vi "Get List Image With Parameters.vi"(0 "Template in":refnum<class "MetaDataObj.lvclass">, 1 "Img Width":u32=230, 3 "DNL_Point":T1={"Horizontal"=-1, "Vertical"=-1}, 5 "Background Color":u32(colorbox)=16777215, 9 "Text Color":u32(colorbox), 11 "error in (no error)":errorcluster, 12 "Highlight?":bool, 13 "Underline Link?":bool) -> (4 "Template out":refnum<class "MetaDataObj.lvclass">, 6 "Image":picture, 10 "End of Desc Character":i32, 14 "Hovering Over Link?":bool, 15 "error out":errorcluster)   [LabVIEW 2016, in "MetaDataObj.lvclass"]
uses:
  <resource>/dialog/NewProjectWizard/MetaDataObj/MetaDataObj.lvclass
  <vilib>/Utility/miscctls.llb/LVPoint32TypeDef.ctl
  <resource>/dialog/NewProjectWizard/MetaDataObj/Accessors/Read Description.vi
  <resource>/dialog/NewProjectWizard/MetaDataObj/Accessors/Read Title.vi
  <resource>/dialog/NewProjectWizard/MetaDataObj/Accessors/Read Icon.vi
  <resource>/dialog/NewProjectWizard/MetaDataObj/Accessors/Read Documentation Path.vi
  <resource>/dialog/NewProjectWizard/MetaDataObj/Accessors/Read Filters.vi
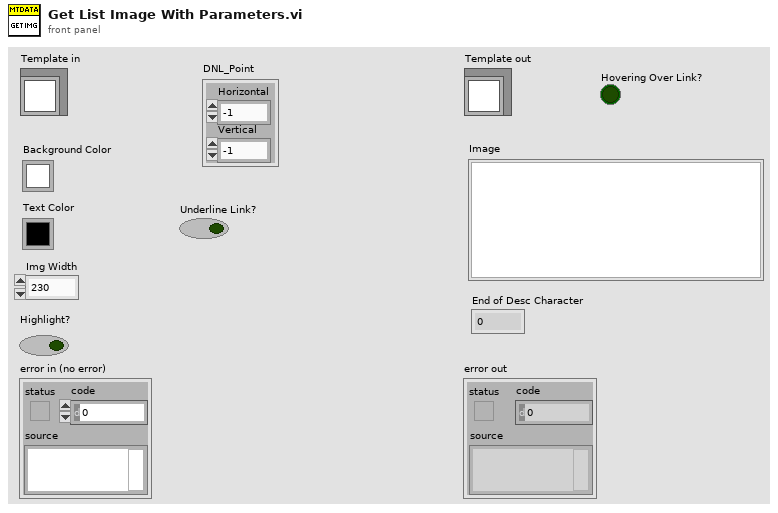
[diagram p1: front panel]
types:
  T1 = typedef "LVPoint32TypeDef.ctl" = cluster{"Horizontal":i32, "Vertical":i32}
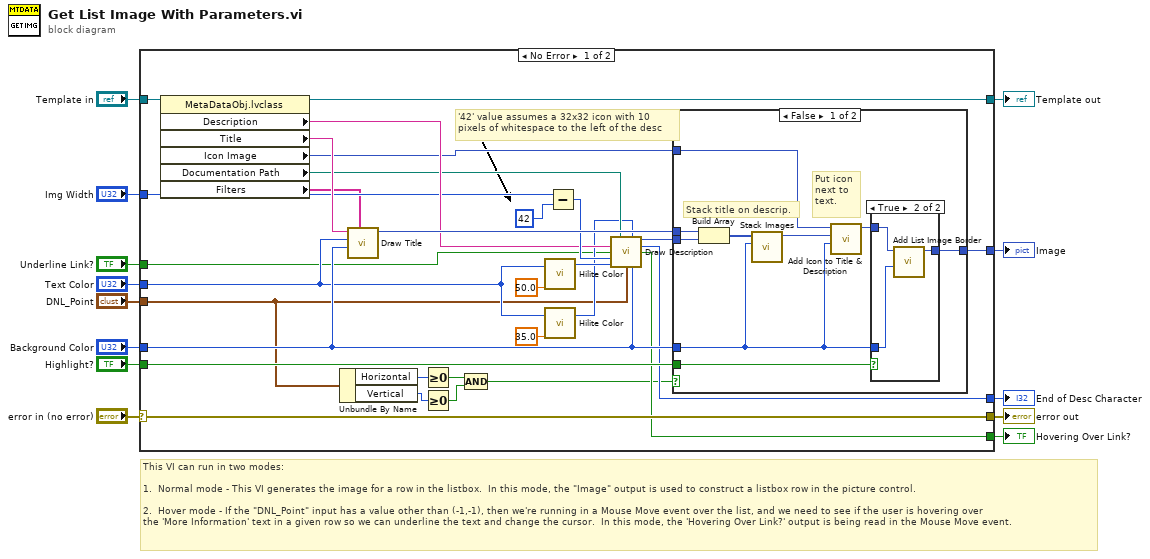
[diagram p0: block diagram]
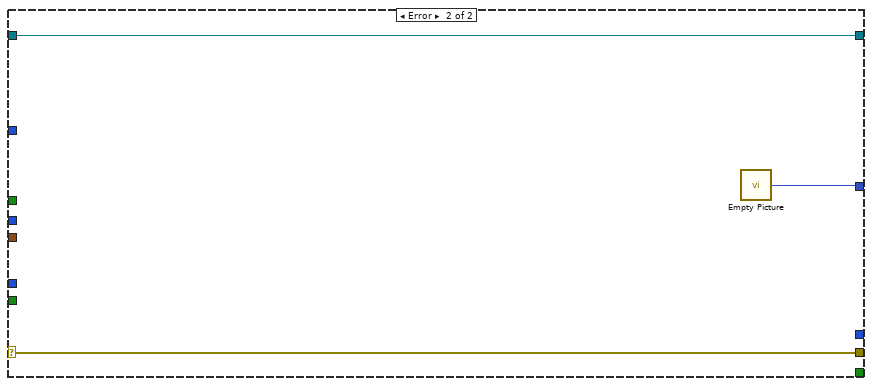
[diagram p4: hidden frame]
diagram:
  # "This VI can run in two modes:\n\n1.  Normal mode - This VI generates the image for a row in the listbox.  In this mode, the \"Image\" output is used to construct a listbox row in the picture control.\n\n2.  Hover mode - If the \"DNL_Point\" input has a value other than (-1,-1), then we're running in a Mouse Move event over the list, and we need to see if the user is hovering over\nthe 'More Information' text in a given row so we can underline the text and change the cursor.  In this mode, the 'Hovering Over Link?' output is being read in the Mouse Move event."
  n1 = case shown="No Error" "error in (no error)" {
    selector: "error in (no error)" -> [w43 w59]
    tunnel: [w43 w59] -> w12
    tunnel: [w33 w58] -> w10
    tunnel: "Template in" -> [w40 w58]
    tunnel: [w36 w57] -> w9
    tunnel: "Img Width" -> [w32 _]
    tunnel: "Text Color" -> [w27 _]
    tunnel: "Background Color" -> [w31 _]
    tunnel: "Highlight?" -> [w30 _]
    tunnel: [w25 _] -> w4
    tunnel: "DNL_Point" -> [w18 _]
    tunnel: [w24 _] -> w2
    tunnel: "Underline Link?" -> [w23 _]
    frame No Error {
      # "'42' value assumes a 32x32 icon with 10\npixels of whitespace to the left of the desc"
      n2 = property class="MetaDataObj.lvclass"(reference=w40) -> (reference out=w33:refnum<class "MetaDataObj.lvclass">, "Description"=w34:string, "Title"=w35:string, "Icon Image"=w15:picture, "Documentation Path"=w29:path, "Filters"=w14:string[])  [unwired: 1 in, 1 out]
      n3 = Unbundle By Name(w18) -> ("Horizontal"=w22:i32, "Vertical"=w21:i32)
      n4 = call <resource>:"Draw Title.vi"("Filters"=w14, "Background Color"=w31, "Text Color"=w27, "Title"=w35) -> ("new picture"=w42:picture)  [unwired: 7 in]
      n5 = Greater Or Equal To 0?(x=w22) -> (x >= 0?=w20:bool)
      n6 = Greater Or Equal To 0?(x=w21) -> (x >= 0?=w19:bool)
      n7 = Compound Arithmetic op=AND(w20, w19) -> (w17:bool)
      n8 = call <vilib>:"Hilite Color.vi"("Percentage(30)"=50.0, "Color In"=w27) -> ("Hilite"=w38:u32)  [unwired: 1 out]
      n9 = call <vilib>:"Hilite Color.vi"("Percentage(30)"=35.0, "Color In"=w27) -> ("Hilite"=w26:u32)  [unwired: 1 out]
      n10 = Subtract(x=w32, y=u32 42 ("x")) -> (x-y=w39:u32)
      n11 = call <resource>:"Draw Description.vi"("DNL_Documentation Path"=w29, "DNL_Link color"=w26, "DNL_String"=w34, "Underline Link?"=w23, "DNL_Word Wrap Bound"=w39, "DNL_Text color"=w38, "DNL_Point"=w18, "DNL_BG color"=w31) -> ("DNL_Image Out"=w41:picture, "End of Desc Character"=w25:i32, "Hovering Over Link?"=w24:bool)  [unwired: 5 in]
      n12 = case shown="False" w17 {
        tunnel: w42 -> [w52 _]
        tunnel: w41 -> [w51 _]
        tunnel: w15 -> [w48 _]
        tunnel: [w47 _] -> w36
        tunnel: w31 -> [w45 _]
        tunnel: w30 -> [w44 _]
        frame False {
          # "Put icon\nnext to\ntext."
          # "Stack title on descrip."
          n13 = Build Array(w52, w51) -> (w50:picture[])
          n14 = call <resource>:"Stack Images.vi"("BG Color"=w45, "Array"=w50) -> ("empty picture"=w49:picture)  [unwired: 9 in]
          n15 = call <resource>:"Add Icon to Title & Description.vi"("Background Color"=w45, "Title & Description"=w49, "Icon"=w48) -> ("Icon + Title & Description"=w46:picture)  [unwired: 8 in]
          n16 = case shown="True" w44 {
            tunnel: [w53 w56] -> w47
            tunnel: w45 -> [_ w55]
            tunnel: w46 -> [w53 w54]
            frame False {
            }
            frame True {
              n17 = call <resource>:"Add List Image Border.vi"("Background Color"=w55, "new picture in"=w54) -> ("new picture out"=w56:picture)  [unwired: 9 in]
            }
          }
        }
        frame True {
          # "Don't need to do any drawing when running\nin Hover mode"
        }
      }
    }
    frame Error {
      n18 = call "Empty Picture"() -> ("empty picture"=w57:picture)
    }
  }
  "error out" <- w12
  "Template out" <- w10
  "Image" <- w9
  "End of Desc Character" <- w4
  "Hovering Over Link?" <- w2
